vi "03-SlideControl.vi"() -> ()   [LabVIEW 2019]
panel:
  out "Gauge":dbl(knob) scale=0.0..10.0
  in  "Slide":dbl(slide) scale=0.0..10.0
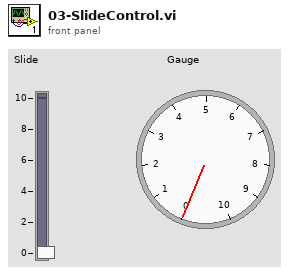
[diagram p1: front panel]
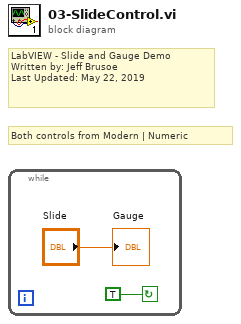
[diagram p0: block diagram]
diagram:
  # "LabVIEW - Slide and Gauge Demo\nWritten by: Jeff Brusoe\nLast Updated: May 22, 2019"
  # "Both controls from Modern | Numeric"
  n1 = while {
    stop <- TRUE continue-if-true
    "Gauge" <- "Slide"
  }
